vi "GetText.vi"(8 "error in":errorcluster, 11 "node in":refnum<class "Dependencies.lvclass">) -> (0 "error out":errorcluster, 1 "additional text":string, 2 "text":string, 3 "node out":refnum<class "Dependencies.lvclass">, 4 "glyph":string)   [LabVIEW 2015, in "Dependencies.lvclass"]
doc: "Returns the text representation of the node used for the tree control.Copyright 2015 National Instruments Corporation\n\nLicensed under the Apache License, Version 2.0 (the \"License\"); you may not use this file except in compliance with the License. You may obtain a copy of the License at http://www.apache.org/licenses/LICENSE-2.0\nUnless required by applicable law or agreed to in writing, software distributed under the License is distributed on an \"AS IS\" BASIS, WITHOUT WARRANTIES OR CONDITIONS OF ANY KIND, either express or implied. See the License for the specific language governing permissions and limitations under the License."
uses:
  Dependencies.lvclass
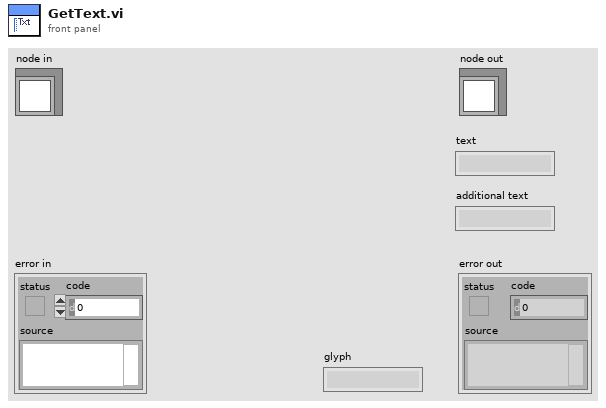
[diagram p1: front panel]
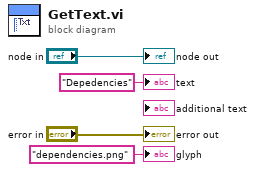
[diagram p0: block diagram]
diagram:
  "error out" <- "error in"
  "node out" <- "node in"
  "text" <- "Depedencies" ("text")
  "glyph" <- "dependencies.png" ("glyph")
